vi "Parse Packet Data (OK).vi"(8 "Error In":errorcluster, 10 "Recieved Bytes":u8[](array[numeric])) -> (0 "Error Out":errorcluster, 2 "Packet Metadata out":T1 {"Server Status" format="%.0x"})   [LabVIEW 2014, in "hse-db.lvlib" / "MySQL (TCP).lvlib"]
uses:
  MySQL (TCP).lvlib
  Controls/OK Packet Metadata.ctl
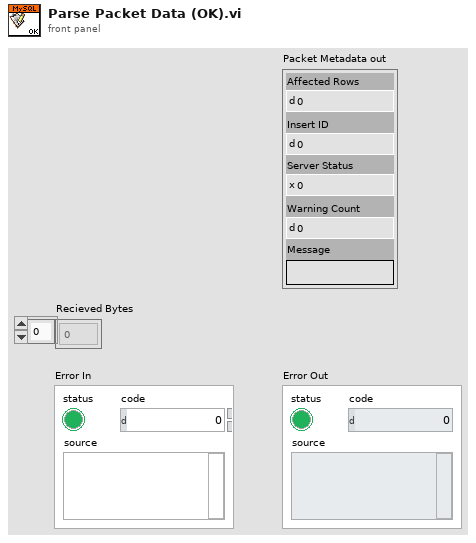
[diagram p1: front panel]
types:
  T1 = typedef "hse-db.lvlib/MySQL (TCP).lvlib/OK Packet Metadata.ctl" = cluster{"Affected Rows":u64, "Insert ID":u64, "Server Status":u16, "Warning Count":u16, "Message":string}
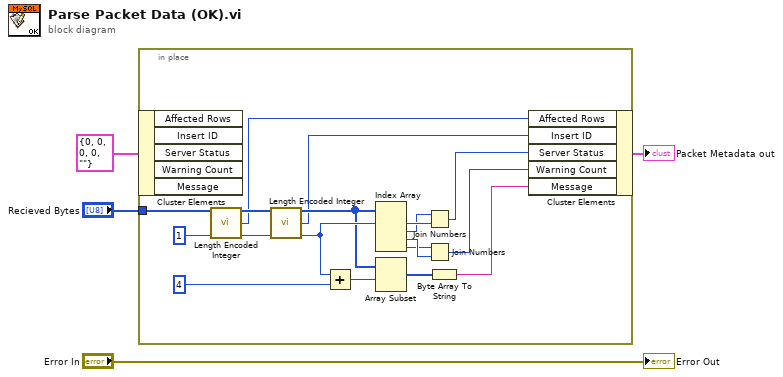
[diagram p0: block diagram]
diagram:
  n1 = in-place {
    in-place-border: "Recieved Bytes" -> [w22]
    n2 = in-place-cluster #1(T1 {"Affected Rows"=0, "Insert ID"=0, "Server Status"=0, "Warning Count"=0, "Message"=""} ("Packet Metadata In")) -> ()  [unwired: 5 out]
    n3 = call "Length Encoded Integer.vi"("Bytes in"=w22, "Start Index(0)"=u64 1 ("Start Index")) -> ("Remaining Bytes out"=w11:u8[], "Integer"=w9:u64, "End Index"=w20:i32)  [unwired: 10 in, 1 out]
    n4 = call "Length Encoded Integer.vi"("Bytes in"=w11, "Start Index(0)"=w20) -> ("Remaining Bytes out"=w10:u8[], "Integer"=w8:u64, "End Index"=w14:i32)  [unwired: 10 in, 1 out]
    n5 = Add(x=w14, y=u64 4) -> (x+y=w15:u64)
    n6 = Index Array(array=w10, index #1=w14) -> (element #1=w19:u8, element #2=w18:u8, element #3=w17:u8, element #4=w16:u8)  [unwired: 3 in]
    n7 = Array Subset(array=w10, index=w15) -> (w12:u8[])  [unwired: 1 in]
    n8 = Join Numbers(hi=w18, lo=w19) -> ((hi.lo)=w7:u16)
    n9 = Join Numbers(hi=w16, lo=w17) -> ((hi.lo)=w6:u16)
    n10 = Byte Array To String(unsigned byte array=w12) -> (string=w5:string)
    n11 = in-place-cluster #1("Affected Rows"=w9, "Insert ID"=w8, "Server Status"=w7, "Warning Count"=w6, "Message"=w5) -> (→"Packet Metadata out":T1)
  }
  "Error Out" <- "Error In"
